vi "generate_front_panel_and_subpanels_controls_dictionary.vi"(9 "additional_language":string, 10 "current_language":string, 11 "main_VI_path":path) -> (2 "all_paths":path[](array[path]), 3 "panels_dictionary_array":string[][](array[string]))   [LabVIEW 2019]
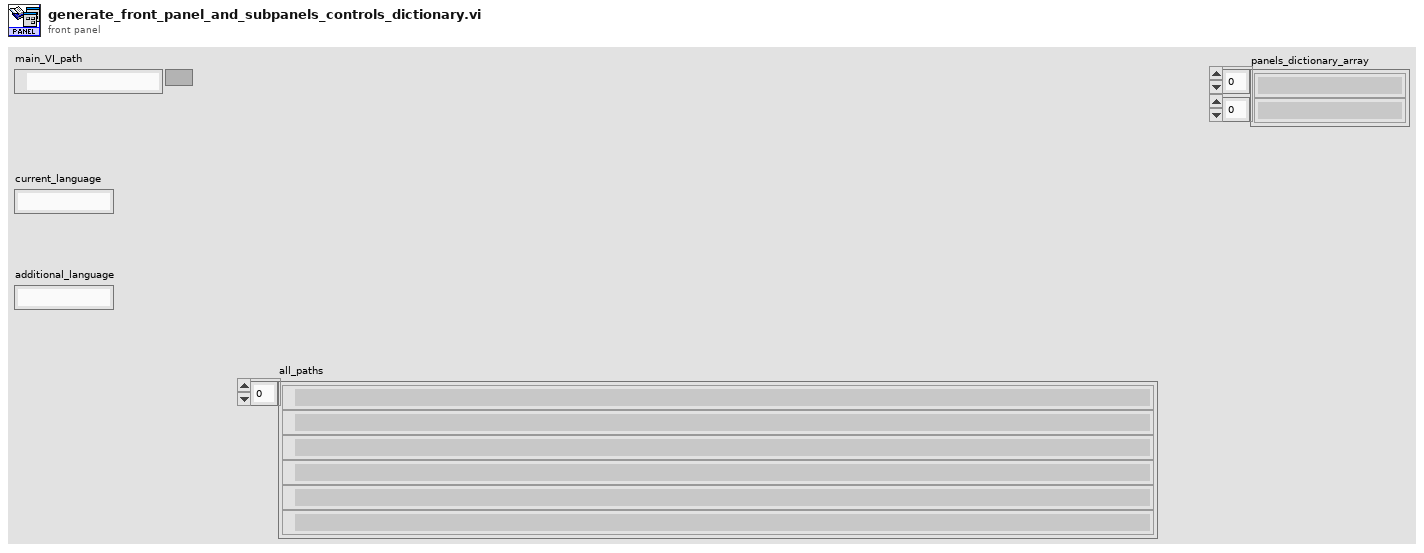
[diagram p1: front panel]
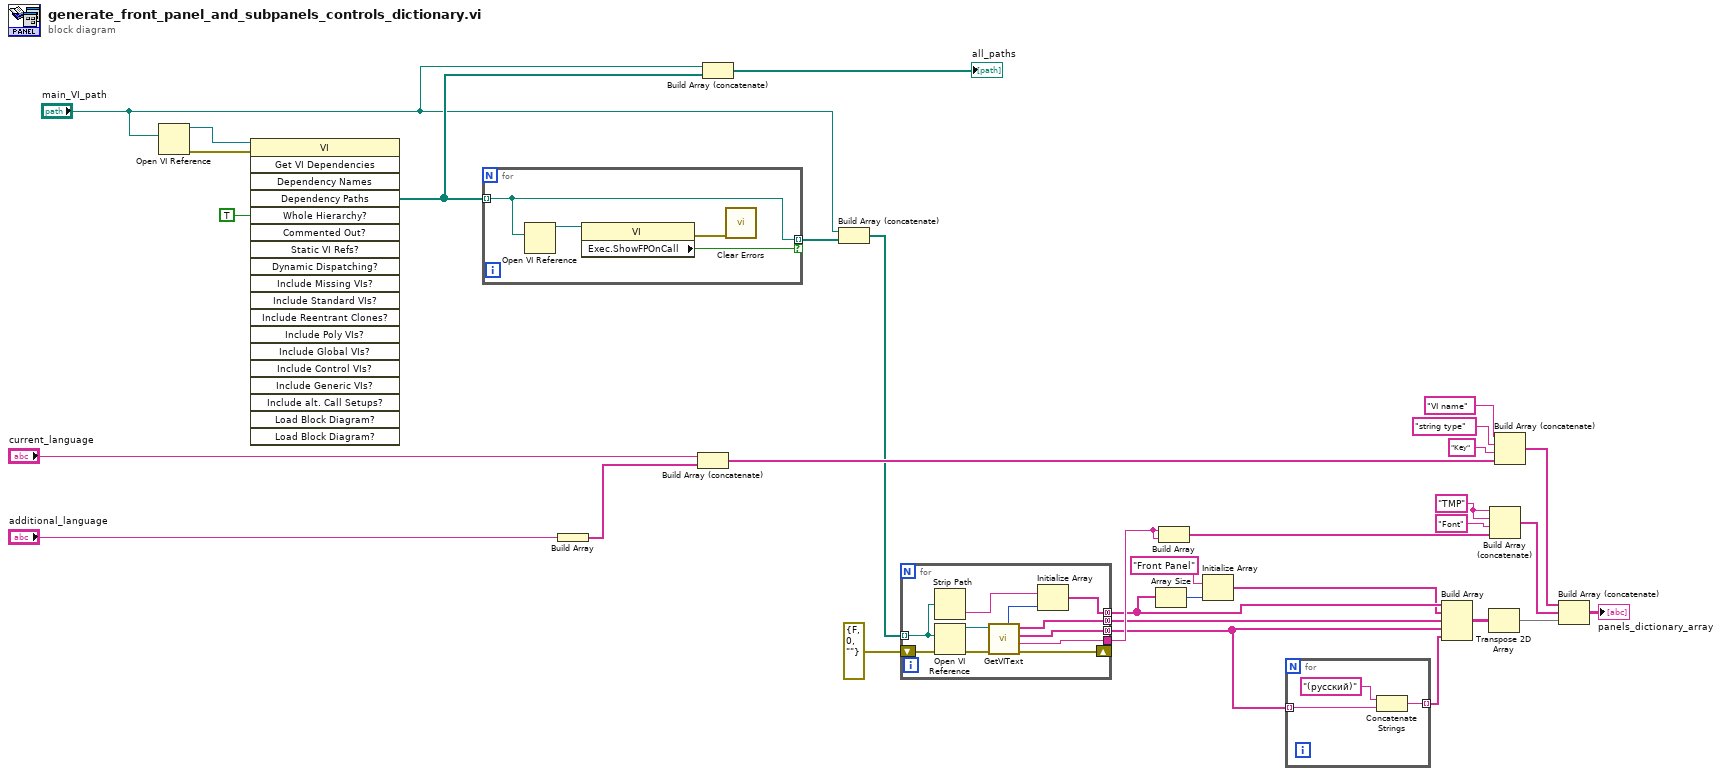
[diagram p0: block diagram]
diagram:
  w9 = "TMP" ("element")
  n1 = Open VI Reference(vi path="main_VI_path") -> (vi reference=w30:refnum<vi>, error out=w29:errorcluster)  [unwired: 5 in]
  n2 = invoke class="VI" method="Get VI Dependencies"(reference=w30, error in=w29, "Whole Hierarchy?"=TRUE) -> ("Dependency Paths"=w12:path[])  [unwired: 16 in, 18 out]
  n3 = for {
    tunnel: w12 -> [w35] mode=indexing
    tunnel: [w35] -> w25 mode=indexing if=w34
    n4 = Open VI Reference(vi path=w35) -> (vi reference=w36:refnum<vi>)  [unwired: 5 in, 1 out]
    n5 = property class="VI"(reference=w36) -> (error out=w33:errorcluster, "Exec.ShowFPOnCall"=w34:bool)  [unwired: 1 in, 1 out]
    n6 = call <vilib>:"Clear Errors.vi"("error in (no error)"=w33) -> ()  [unwired: 5 in, 2 out]
  }
  n7 = Build Array("additional_language") -> (w32:string[])
  n8 = Build Array (concatenate)("current_language", w32) -> (w19:string[])
  n9 = Build Array (concatenate)("main_VI_path", w12) -> (→"all_paths":path[])
  n10 = Build Array (concatenate)("main_VI_path", w25) -> (w13:path[])
  n11 = for {
    tunnel: w13 -> [w41] mode=indexing
    tunnel: [w47] -> w2 mode=concatenating
    tunnel: [w40] -> w14 mode=concatenating
    shift-right: [w46] -> _
    shift-left: errorcluster {"status"=FALSE, "code"=0, "source"=""} ("error in (no error)") -> [w44]
    tunnel: [w45] -> w16
    tunnel: [w37] -> w4 mode=concatenating
    n12 = Strip Path(path=w41) -> (name=w38:string)  [unwired: 1 out]
    n13 = Open VI Reference(vi path=w41, error in (no error)=w44) -> (vi reference=w42:refnum<vi>, error out=w43:errorcluster)  [unwired: 4 in]
    n14 = call "GetVIText.vi"("error in (no error)"=w43, "VI"=w42) -> ("error out"=w46:errorcluster, "Font Name"=w45:string, "Control Text"=w47:string[], "Control Keys"=w40:string[], "number_of_records"=w39:i32)  [unwired: 5 in]
    n15 = Initialize Array(w38, w39) -> (w37:string[])
  }
  n16 = Array Size(array=w4) -> (size(s)=w8:i32)
  n17 = Build Array(w16, w16) -> (w15:string[])
  n18 = Initialize Array("Front Panel" ("element"), w8) -> (w3:string[])
  n19 = for {
    tunnel: w2 -> [w49] mode=indexing
    tunnel: [w48] -> w1 mode=indexing
    n20 = Concatenate Strings("(русский)", w49) -> (w48:string)
  }
  n21 = Build Array(w4, w3, w14, w2, w1) -> (w18:string[][])
  n22 = Transpose 2D Array(2D array=w18) -> (transposed array=w17:string[][])
  n23 = Build Array (concatenate)(w9, w9, "Font", w15) -> (w21:string[])
  n24 = Build Array (concatenate)("VI name" ("element"), "string type" ("element"), "Key", w19) -> (w24:string[])
  n25 = Build Array (concatenate)(w24, w21, w17) -> (→"panels_dictionary_array":string[][])
